vi "Initialize Monitors.vi"(8 "error in":errorcluster, 10 "channel number":u8, 11 "board handle":u8) -> (0 "error out":errorcluster, 2 "channel number out":u8, 3 "board handle out":u8)   [LabVIEW 2020, in "AIM ARINC 429 Hardware API.lvlib"]
uses:
  AIM ARINC 429 Hardware API.lvlib
  <instrlib>/AIM GmbH/_ARINC-429/AIM429LV.lvlib
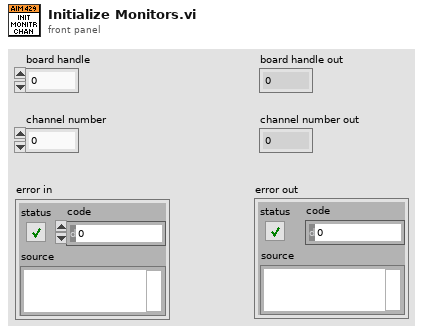
[diagram p1: front panel]
types:
  T1 = cluster{"mode":i32, "size_in_entries":u32, "tat_count":u32, "interrupt_mode":i32}
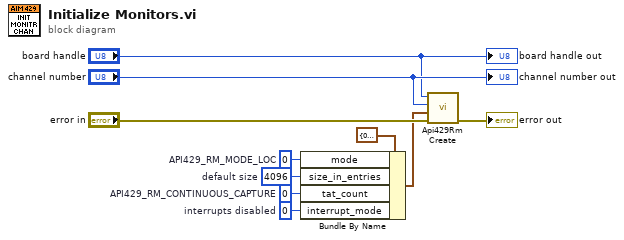
[diagram p0: block diagram]
diagram:
  w2 = 0  # API429_RM_MODE_LOC
  w3 = u32 4096  # default size
  w4 = 0  # interrupts disabled
  w5 = u32 0  # API429_RM_CONTINUOUS_CAPTURE
  n1 = Bundle By Name(cluster=T1 {"mode"=0, "size_in_entries"=0, "tat_count"=0, "interrupt_mode"=0} ("setup"), "mode"=w2, "size_in_entries"=w3, "tat_count"=w5, "interrupt_mode"=w4) -> (w1:T1)
  n2 = call <instrlib>:"Api429Rm Create.vi"("error in (no error)"="error in", "setup"=w1, "channel_id"="channel number", "board_handle"="board handle") -> ("error out"=→"error out":errorcluster)  [unwired: 7 in]
  "board handle out" <- "board handle"
  "channel number out" <- "channel number"
